vi "Get Discovery Service Address.vi"(8 "error in":errorcluster, 11 "cluster id":string) -> (0 "error out":errorcluster, 3 "address":string)   [LabVIEW 2021, in "NI Measurement Plug-In SDK.lvlib"]
doc: "This VI is deprecated. Please use <b>NI Discovery V1 Client::Get Discovery Service Address.vi</b> for the same functionality."
uses:
  NI Measurement Plug-In SDK.lvlib
  Clients/Discovery V1/NI Discovery V1 Client.lvlib
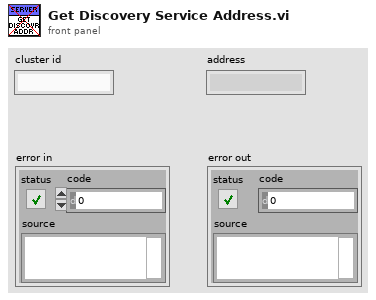
[diagram p1: front panel]
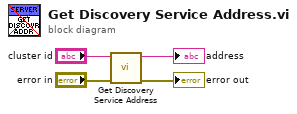
[diagram p0: block diagram]
diagram:
  n1 = call "Get Discovery Service Address.vi"("error in"="error in", "cluster id (\"\")"="cluster id") -> ("error out"=→"error out":errorcluster, "address"=→"address":string)  [unwired: 8 in]
